vi "MPExxx_set_ovp_ocp.vi"(2 "error in (no error)":errorcluster, 3 "Set OCP":dbl format="%.2f", 4 "Set OVP":dbl format="%.2f", 5 "VISA session":refnum<visa-resource-name>) -> (0 "error out":errorcluster, 1 "dup VISA session":refnum<visa-resource-name>)   [LabVIEW 2017]
doc: "This form sets the over-voltage and over-current protection set points."
panel:
  # "MAGNA-POWER"
  # "Electronics"
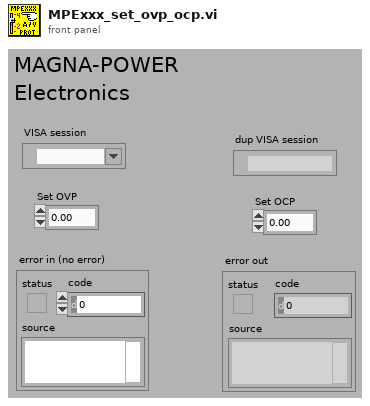
[diagram p1: front panel]
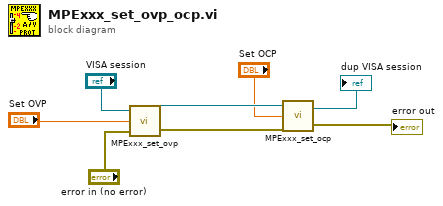
[diagram p0: block diagram]
diagram:
  n1 = call "MPExxx_set_ovp.vi"("error in (no error)"="error in (no error)", "Set OVP"="Set OVP", "VISA session"="VISA session") -> ("error out"=w8:errorcluster, "dup VISA session"=w7:refnum<visa-resource-name>)
  n2 = call "MPExxx_set_ocp.vi"("error in (no error)"=w8, "Set OCP"="Set OCP", "VISA session"=w7) -> ("error out"=→"error out":errorcluster, "dup VISA session"=→"dup VISA session":refnum<visa-resource-name>)
